vi "Top-Level VI.vi"() -> ()   [LabVIEW 2010, in "TS Simple LabVIEW OI.lvlib"]
uses:
  TS Simple LabVIEW OI.lvlib
  TS Simple LabVIEW OI Dependencies.lvlib
panel:
  in  "Terminate All Button":refnum<k7>(container)
  in  "Exit Button":refnum<k7>(container)
  in  "Login/Logout Button":refnum<k7>(container)
  in  "Close Executions Button":refnum<k7>(container)
  in  "Break/Resume Button":refnum<k7>(container)
  in  "Terminate/Restart Button":refnum<k7>(container)
  in  "Run Selected Sequence Button":refnum<k7>(container)
  in  "Entry Point 2 Button":refnum<k7>(container)
  in  "Entry Point 1 Button":refnum<k7>(container)
  in  "Report Viewer":refnum<k7>(container)
  in  "Close Sequence File Button":refnum<k7>(container)
  in  "Open Sequence File Button":refnum<k7>(container)
  in  "Executions ComboBox":refnum<k7>(container) caption="Executions:"
  in  "Sequences ComboBox":refnum<k7>(container) caption="Sequences:"
  in  "Execution View":refnum<k7>(container)
  in  "Sequence Files ComboBox":refnum<k7>(container) caption="Sequence Files:"
  in  "ExecutionView Manager":refnum<k7>(container)
  in  "SequenceFileView Manager":refnum<k7>(container)
  in  "Application Manager":refnum<k7>(container)
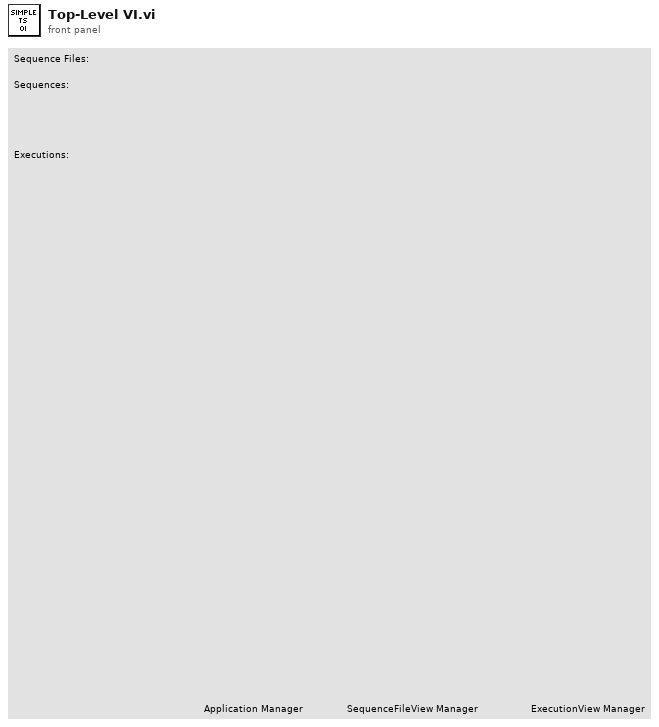
[diagram p1: front panel]
types:
  T1 = enum32{"invalid app kind", "Development System", "Run Time System", "Student Edition", "Embedded LabVIEW", "Evaluation", "Custom"}
  T2 = cluster{"Login/Logout Button":refnum<k7>, "Exit Button":refnum<k7>, "Terminate All Button":refnum<k7>}
  T3 = cluster{"Sequence Files ComboBox":refnum<k7>, "Sequences ComboBox":refnum<k7>, "Open Sequence File Button":refnum<k7>, "Close Sequence File Button":refnum<k7>, "Entry Point 1 Button":refnum<k7>, "Entry Point 2 Button":refnum<k7>, "Run Selected Sequence Button":refnum<k7>}
  T4 = cluster{"Executions ComboBox":refnum<k7>, "Execution View":refnum<k7>, "Report Viewer":refnum<k7>, "Close Executions Button":refnum<k7>, "Break/Resume Button":refnum<k7>, "Terminate/Restart Button":refnum<k7>}
  T5 = cluster{"Quit Application Event":refnum<user-event>, refnum<vi>, "ExecutionView Manager":refnum<k7>, "SequenceFileView Manager":refnum<k7>}
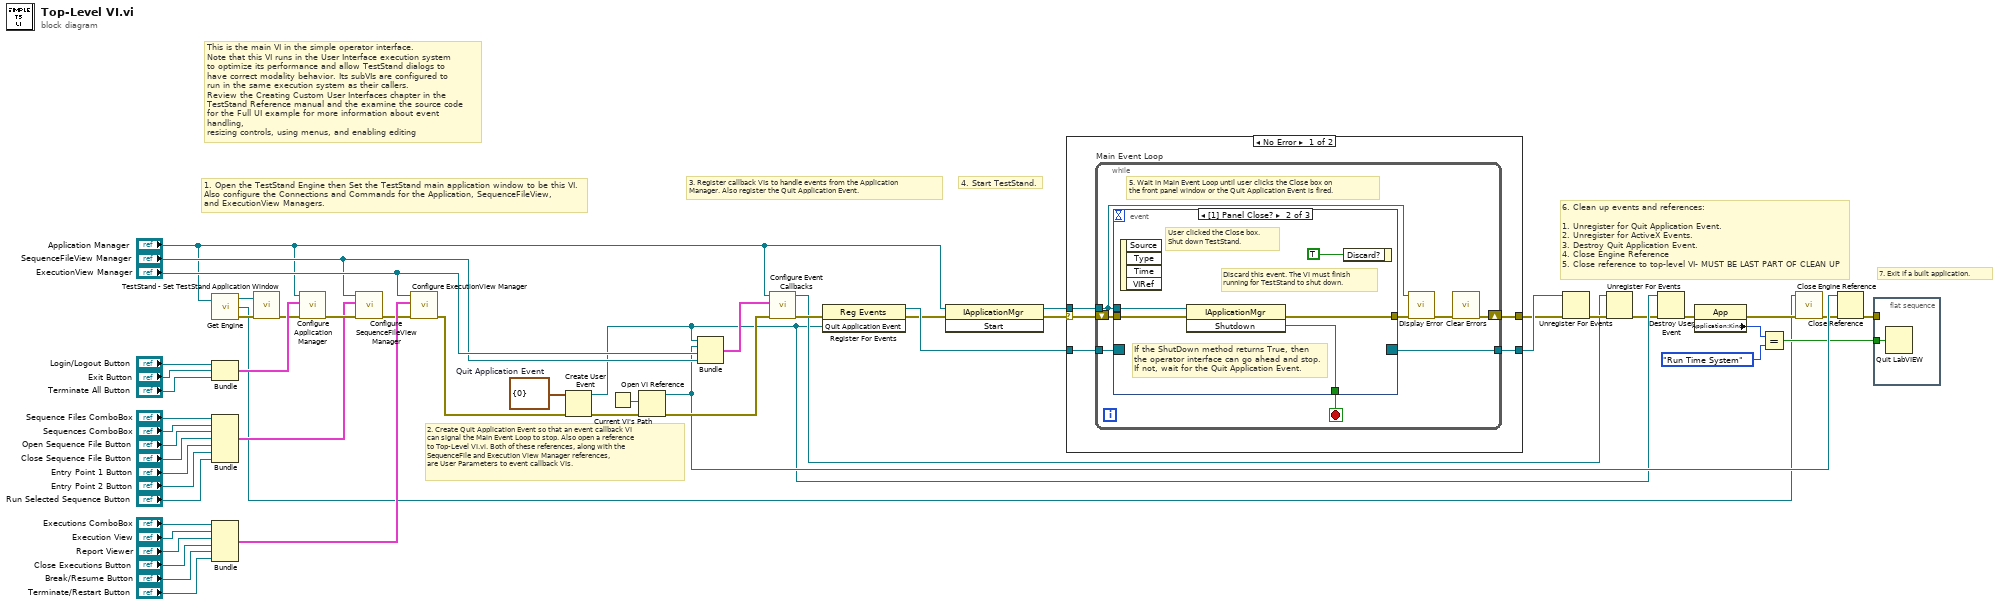
[diagram p0: block diagram]
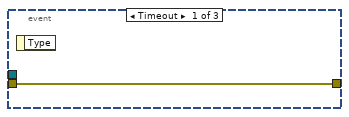
[diagram p2: hidden frame]
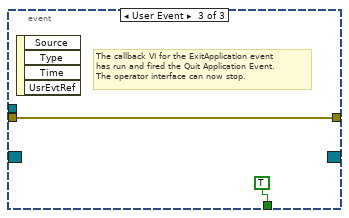
[diagram p3: hidden frame]
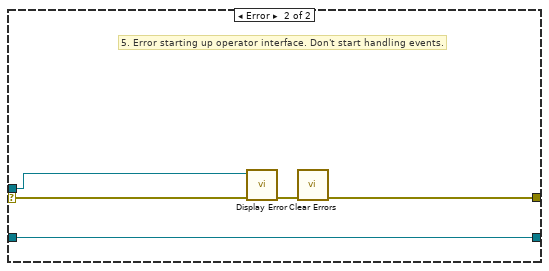
[diagram p4: hidden frame]
diagram:
  w52 = cluster{"Number":i32} {"Number"=0}  # Quit Application Event
  # "This is the main VI in the simple operator interface.\nNote that this VI runs in the User Interface execution system\nto optimize its performance and allow TestStand dialogs to\nhave correct modality behavior. Its subVIs are configured to\nrun in the same execution system as their callers.\nReview the Creating Custom User Interfaces chapter in the \nTestStand Reference manual and the examine the source code\nfor the Full UI example for more information about event handling,\nresizing controls, using menus, and enabling editing"
  # "7. Exit if a built application."
  # "4. Start TestStand."
  # "3. Register callback VIs to handle events from the Application\nManager. Also register the Quit Application Event."
  # "2. Create Quit Application Event so that an event callback VI\ncan signal the Main Event Loop to stop. Also open a reference\nto Top-Level VI.vi. Both of these references, along with the\nSequenceFile and Execution View Manager references,\nare User Parameters to event callback VIs."
  # "6. Clean up events and references:\n\n1. Unregister for Quit Application Event.\n2. Unregister for ActiveX Events.\n3. Destroy Quit Application Event.\n4. Close Engine Reference\n5. Close reference to top-level VI- MUST BE LAST PART OF CLEAN UP"
  # "1. Open the TestStand Engine then Set the TestStand main application window to be this VI. \nAlso configure the Connections and Commands for the Application, SequenceFileView, \nand ExecutionView Managers."
  n1 = call "Get Engine.vi"("Application Manager In"="Application Manager") -> ("Application Manager Out"=w4:refnum<k7>, "TestStand Engine"=w2:refnum<k7>, "error out"=w6:errorcluster)  [unwired: 1 in]
  n2 = Bundle("Login/Logout Button"="Login/Logout Button", "Exit Button"="Exit Button", "Terminate All Button"="Terminate All Button") -> (w17:T2)  [unwired: 1 out]
  n3 = Bundle("Sequence Files ComboBox"="Sequence Files ComboBox", "Sequences ComboBox"="Sequences ComboBox", "Open Sequence File Button"="Open Sequence File Button", "Close Sequence File Button"="Close Sequence File Button", "Entry Point 1 Button"="Entry Point 1 Button", "Entry Point 2 Button"="Entry Point 2 Button", "Run Selected Sequence Button"="Run Selected Sequence Button") -> (w12:T3)  [unwired: 1 out]
  n4 = Bundle("Executions ComboBox"="Executions ComboBox", "Execution View"="Execution View", "Report Viewer"="Report Viewer", "Close Executions Button"="Close Executions Button", "Break/Resume Button"="Break/Resume Button", "Terminate/Restart Button"="Terminate/Restart Button") -> (w31:T4)  [unwired: 1 out]
  n5 = call <vilib>:"TestStand - Set TestStand Application Window.vi"("error in (no error)"=w6, "Application Manager"=w4) -> ("error out"=w10:errorcluster)  [unwired: 1 in, 8 out]
  n6 = call "Configure Application Manager.vi"("error in (no error)"=w10, "UI Control References"=w17, "Application Manager"="Application Manager") -> ("error out"=w20:errorcluster)  [unwired: 8 out]
  n7 = call "Configure SequenceFileView Manager.vi"("error in (no error)"=w20, "UI Control References"=w12, "SequenceFileView Manager"="SequenceFileView Manager") -> ("error out"=w30:errorcluster)  [unwired: 7 in, 1 out]
  n8 = call "Configure ExecutionView Manager.vi"("error in (no error)"=w30, "UI Control References"=w31, "ExecutionView Manager"="ExecutionView Manager") -> ("error out"=w7:errorcluster)  [unwired: 5 in, 3 out]
  n9 = Create User Event(user event datatype=w52, error in=w7) -> (user event=w21:refnum<user-event>, error out=w27:errorcluster)
  n10 = Current VI's Path() -> (path=w50:path)
  n11 = Open VI Reference(vi path=w50, error in (no error)=w27) -> (vi reference=w22:refnum<vi>, error out=w26:errorcluster)  [unwired: 4 out]
  n12 = Bundle("Quit Application Event"=w21, w22, "ExecutionView Manager"="ExecutionView Manager", "SequenceFileView Manager"="SequenceFileView Manager") -> (w28:T5)  [unwired: 1 out]
  n13 = call "Configure Event Callbacks.vi"("error in (no error)"=w26, "User Parameters"=w28, "Application Manager"="Application Manager") -> ("error out"=w25:errorcluster, "Event Callback Refnum Out"=w23:refnum<k27>)  [unwired: 4 in, 3 out]
  n14 = register-events(error in=w25, w21) -> (reference out=w53:refnum<event-registration>, error out=w49:errorcluster)  [unwired: 1 in]
  n15 = invoke class="IApplicationMgr" method="Start"(reference="Application Manager", error in=w49) -> (reference out=w51:refnum<k7>, error out=w48:errorcluster)  [unwired: 1 in, 1 out]
  n16 = case shown="No Error" w48 {
    selector: w48 -> [w55 w77]
    tunnel: w53 -> [w58 w79]
    tunnel: [w57 w79] -> w47
    tunnel: w51 -> [w56 w76]
    tunnel: [w54 w78] -> w46
    frame No Error {
      n17 = while "Main Event Loop" {
        tunnel: w58 -> [w65]
        tunnel: [w64] -> w57
        shift-right: [w60] -> w54
        shift-left: w55 -> [w63]
        tunnel: w56 -> [w59]
        stop <- w66 stop-if-true
        # "5. Wait in Main Event Loop until user clicks the Close box on\nthe front panel window or the Quit Application Event is fired."
        n18 = event shown="[1] Panel Close?" {
          selector: w65 -> [_ _ _]
          dyn-events: [_ _ _] -> w64
          timeout: _ -> [_ _ _]
          tunnel: w59 -> [_ w71 _]
          tunnel: w63 -> [w67 w72 w73]
          tunnel: [_ w70 TRUE ("ShutDown")] -> w66
          tunnel: [w67 w69 w73] -> w62
          event Timeout {
            n19 = event-data() -> ()  [unwired: 2 out]
          }
          event Panel Close? {
            # "Discard this event. The VI must finish\nrunning for TestStand to shut down."
            # "If the ShutDown method returns True, then\nthe operator interface can go ahead and stop.\nIf not, wait for the Quit Application Event."
            # "User clicked the Close box.\nShut down TestStand."
            n20 = event-data() -> ()  [unwired: 5 out]
            n21 = invoke class="IApplicationMgr" method="Shutdown"(reference=w71, error in=w72) -> (error out=w69:errorcluster, "Shutdown"=w70:bool)  [unwired: 1 in, 1 out]
            n22 = event-data("Discard?"=TRUE) -> ()  [unwired: 1 in, 1 out]
          }
          event User Event {
            # "The callback VI for the ExitApplication event\nhas run and fired the Quit Application Event.\nThe operator interface can now stop."
            n23 = event-data() -> ()  [unwired: 5 out]
          }
        }
        n24 = call "Display Error.vi"("error in (no error)"=w62, "Application Manager"=w59) -> ("error out"=w61:errorcluster)  [unwired: 9 out]
        n25 = call <vilib>:"Clear Errors.vi"("error in (no error)"=w61) -> ("error out"=w60:errorcluster)  [unwired: 6 out]
      }
    }
    frame Error {
      # "5. Error starting up operator interface. Don't start handling events."
      n26 = call "Display Error.vi"("error in (no error)"=w77, "Application Manager"=w76) -> ("error out"=w75:errorcluster)  [unwired: 9 out]
      n27 = call <vilib>:"Clear Errors.vi"("error in (no error)"=w75) -> ("error out"=w78:errorcluster)  [unwired: 6 out]
    }
  }
  n28 = Unregister For Events(event registration refnum=w47, error in=w46) -> (error out=w45:errorcluster)
  n29 = Unregister For Events(event registration refnum=w23, error in=w45) -> (error out=w9:errorcluster)
  n30 = Destroy User Event(user event=w21, error in=w9) -> (error out=w16:errorcluster)
  n31 = property class="App"(error in=w16) -> (error out=w3:errorcluster, "Application:Kind"=w15:T1)  [unwired: 1 in, 1 out]
  n32 = Equal?(x=w15, y=T1."Run Time System" ("Application:Kind")) -> (x = y?=w13:bool)
  n33 = call "Close Engine Reference.vi"("error in (no error)"=w3, "TestStand Engine"=w2) -> ("error out"=w1:errorcluster)  [unwired: 1 in, 8 out]
  n34 = Close Reference(reference=w22, error in (no error)=w1) -> (error out=w8:errorcluster)
  n35 = flat-sequence {
    tunnel: w13 -> [w80]
    tunnel: w8 -> [_]
    frame #0 {
      n36 = Quit LabVIEW(quit? (T)=w80) -> ()
    }
  }
